vi "Servo MSMT Set Servo Type in Measurement Name.vi"(8 "error in (no error)":errorcluster, 11 "Servo to Compression in":refnum<class "Servo to Compression.lvclass">) -> (0 "error out":errorcluster, 3 "Servo to Compression out":refnum<class "Servo to Compression.lvclass">)   [LabVIEW 2018, in "Servo to Compression.lvlib" / "Servo to Compression.lvclass"]
uses:
  Servo to Compression.lvclass
  C:/Sequence Automation/Plugins/Measurement Interface.lvlibp/Measurement Interface.lvclass
  Plugins/Measurement Interface.lvlibp/Private Methods/Measurement Name/Read Measurement Name.vi
  Plugins/Measurement Interface.lvlibp/Private Methods/Measurement Name/Write Measurement Name.vi
  Plugins/Measurements/Servo MSMT.lvlibp/Servo MSMT.lvclass
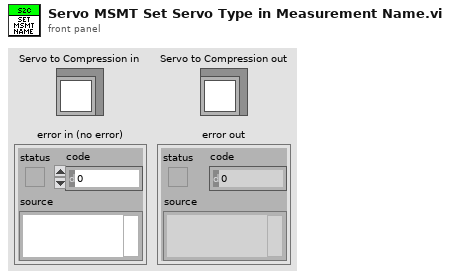
[diagram p1: front panel]
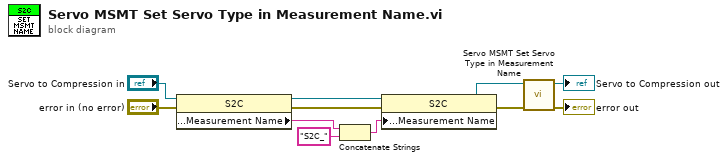
[diagram p0: block diagram]
diagram:
  n1 = property class="S2C"(reference="Servo to Compression in", error in="error in (no error)") -> (reference out=w3:refnum<class "Servo to Compression.lvclass">, error out=w10:errorcluster, "Public Methods:Measurement Name"=w9:string)
  n2 = Concatenate Strings(w9, "S2C_" ("string")) -> (w1:string)
  n3 = property class="S2C"(reference=w3, error in=w10, "Public Methods:Measurement Name"=w1) -> (reference out=w2:refnum<class "Servo to Compression.lvclass">, error out=w4:errorcluster)
  n4 = call-parent "Servo MSMT Set Servo Type in Measurement Name.vi"("error in (no error)"=w4, "Servo MSMT in"=w2) -> ("error out"=→"error out":errorcluster, "Servo MSMT out"=→"Servo to Compression out":refnum<class "Servo to Compression.lvclass">)  [unwired: 8 in]
